vi "getGrating.vi"(11 "VISA":refnum<visa-resource-name>) -> (2 "gratingOut":i32, 3 "VISAOUT":refnum<visa-resource-name>)   [LabVIEW 2018]
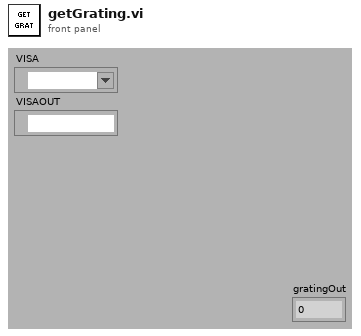
[diagram p1: front panel]
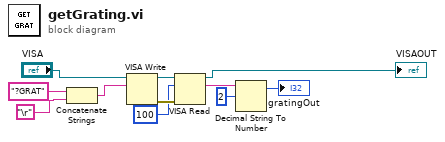
[diagram p0: block diagram]
diagram:
  n1 = Concatenate Strings("?GRAT", "\r") -> (w5:string)
  n2 = VISA Write(VISA resource name="VISA", write buffer=w5) -> (VISA resource name out=w4:refnum<visa-resource-name>, error out=w10:errorcluster)  [unwired: 1 in, 1 out]
  n3 = VISA Read(VISA resource name=w4, byte count=u32 100, error in (no error)=w10) -> (VISA resource name out=→"VISAOUT":refnum<visa-resource-name>, read buffer=w8:string)  [unwired: 2 out]
  n4 = Decimal String To Number(string=w8, offset=2) -> (offset past number=→"gratingOut":i32)  [unwired: 1 in, 1 out]
